vi "Init Messaging.vi"(8 "error in (no error)":errorcluster, 10 "Server Host":string, 11 "LV Chat Client in":refnum<class "LV Chat Client.lvclass">) -> (0 "error out":errorcluster, 3 "LV Chat Client out":refnum<class "LV Chat Client.lvclass">)   [LabVIEW 2020, in "LV Chat Client.lvclass"]
uses:
  LV Chat Client.lvclass
  <vilib>/IlluminatedG/lv-stream-tcp/TCP Client/TCP Client.lvclass
  C:/Program Files (x86)/National Instruments/LabVIEW 2020/vi.lib/IlluminatedG/lv-stream/Endpoint/Endpoint.lvclass
  <vilib>/IlluminatedG/lv-stream/URI/URI.lvclass
  Data Types/Message ID.ctl
  LV Chat Client.lvclass/LV Chat Client.ctl
  53c0471a-ae57-4e0d-849a-9e110c4ef324.vi
  bfa1ed70-9715-4b9c-a241-1f960be845c7.vi
  5a9cbe4e-b617-4434-a5f9-4db64dc2f399.vi
  User Info Message Callback.vi
  Userlist Message Callback.vi
  Chat Message Callback.vi
  Connection Callback.vi
  <vilib>/IlluminatedG/lv-stream/Endpoint/Endpoint.lvclass
  Stream-Simple-Msg/Manager/Manager.lvclass
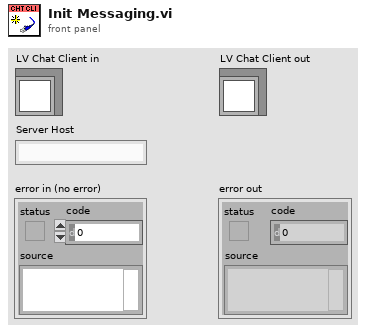
[diagram p1: front panel]
types:
  T1 = typedef "Message ID.ctl" = enum16{"UserInfo", "UserList", "Message", "Disconnect"}
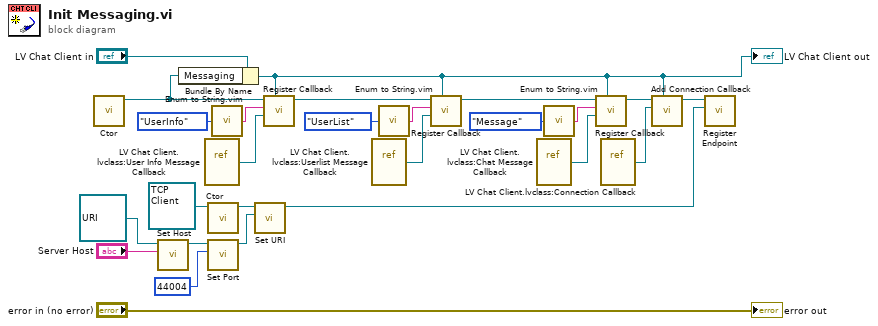
[diagram p0: block diagram]
diagram:
  n1 = call "Ctor.vi"() -> ("Manager out"=w17:refnum<class "Manager.lvclass">)  [unwired: 10 in, 1 out]
  n2 = call <vilib>:"Set Host.vi"("Host"="Server Host", "URI in"=refnum<class "URI.lvclass"> refnum) -> ("URI out"=w22:refnum<class "URI.lvclass">)  [unwired: 8 in, 1 out]
  n3 = Bundle By Name(cluster="LV Chat Client in", "Messaging"=w17) -> (w2:refnum<class "LV Chat Client.lvclass">)
  "LV Chat Client out" <- w2
  n4 = vi-ref "LV Chat Client.lvclass:User Info Message Callback.vi"() -> (w14:refnum<vi>)
  n5 = call-dynamic "Ctor.vi"("TCP Client in"=refnum<class "TCP Client.lvclass"> refnum ("Stream-TCP.lvlib:TCP Client.lvclass")) -> ("TCP Client out"=w20:refnum<class "TCP Client.lvclass">)  [unwired: 9 in, 1 out]
  n6 = call <vilib>:"Set Port.vi"("Port"=u16 44004, "URI in"=w22) -> ("URI out"=w19:refnum<class "URI.lvclass">)  [unwired: 8 in, 1 out]
  n7 = call "Enum to String.vim"("Enum"=Message_ID."UserInfo" ("Message ID")) -> ("Enum String"=w15:string)
  n8 = call <vilib>:"Set URI.vi"("URI"=w19, "Endpoint in"=w20) -> ("Endpoint out"=w5:refnum<class "TCP Client.lvclass">)  [unwired: 8 in, 1 out]
  n9 = call "Register Callback.vi"("Owner"=w2, "Callback"=w14, "Message ID"=w15, "Manager in"=w17) -> ("Manager out"=w10:refnum<class "Manager.lvclass">)  [unwired: 6 in, 1 out]
  n10 = vi-ref "LV Chat Client.lvclass:Userlist Message Callback.vi"() -> (w13:refnum<vi>)
  n11 = call "Enum to String.vim"("Enum"=Message_ID."UserList" ("Message ID")) -> ("Enum String"=w12:string)
  n12 = call "Register Callback.vi"("Owner"=w2, "Callback"=w13, "Message ID"=w12, "Manager in"=w10) -> ("Manager out"=w6:refnum<class "Manager.lvclass">)  [unwired: 6 in, 1 out]
  n13 = vi-ref "LV Chat Client.lvclass:Chat Message Callback.vi"() -> (w7:refnum<vi>)
  n14 = call "Enum to String.vim"("Enum"=Message_ID."Message" ("Message ID")) -> ("Enum String"=w8:string)
  n15 = call "Register Callback.vi"("Owner"=w2, "Callback"=w7, "Message ID"=w8, "Manager in"=w6) -> ("Manager out"=w4:refnum<class "Manager.lvclass">)  [unwired: 6 in, 1 out]
  n16 = vi-ref "LV Chat Client.lvclass:Connection Callback.vi"() -> (w1:refnum<vi>)
  n17 = call "Add Connection Callback.vi"("Owner"=w2, "Callback"=w1, "Manager in"=w4) -> ("Manager out"=w3:refnum<class "Manager.lvclass">)  [unwired: 7 in, 1 out]
  n18 = call "Register Endpoint.vi"("Stream:Endpoint"=w5, "Manager in"=w3) -> ()  [unwired: 8 in, 2 out]
  "error out" <- "error in (no error)"
